vi "SendSignal.vi"(11 "Signal":T1) -> ()   [LabVIEW 2011]
uses:
  Signal.ctl
  SignalAction.ctl
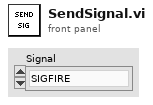
[diagram p1: front panel]
types:
  T1 = typedef "Signal.ctl" = enum16{"SIGFIRE", "SIGSTOPSCRIPT", "SIGSTARTGUN", "SIGSTOPGUN", "SIGDISABLED", "SIGENABLED", "SIGUDPTIMEOUT", "SIGNEWVISION_REMOTE", "SIGNEWVISION_LOCAL", "SIGSHOTFIRED", "SIGDOTRACK", "SIGDONTTRACK"}
  T2 = typedef "SignalAction.ctl" = enum16{"Send Signal", "Get Signal Trap"}
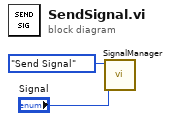
[diagram p0: block diagram]
diagram:
  n1 = call "SignalManager.vi"("Signal"="Signal", "Signal Action"=SignalAction."Send Signal") -> ()  [unwired: 9 in, 1 out]
